vi "Create Object.vi"() -> (3 "LVCAM Destroy Self Msg out":refnum<class "LVCAM Destroy Self Msg.lvclass">)   [LabVIEW 2021, in "LVCAM Destroy Self.lvlib" / "LVCAM Destroy Self Msg.lvclass"]
uses:
  LVCAM Destroy Self Msg.lvclass
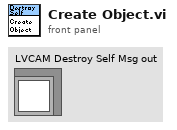
[diagram p1: front panel]
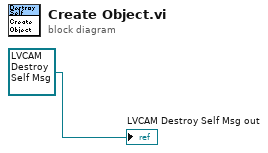
[diagram p0: block diagram]
diagram:
  "LVCAM Destroy Self Msg out" <- refnum<class "LVCAM Destroy Self Msg.lvclass"> refnum ("Destroy Msg in")
